vi "Event Handle Loop_Initialize.vi"(8 "error in (no error)":errorcluster, 11 "QMenu Class in":refnum<class "QMenu Class.lvclass">) -> (0 "error out":errorcluster, 3 "QMenu Class out":refnum<class "QMenu Class.lvclass">)   [LabVIEW 2020, in "QTab.lvlib" / "QMenu Class.lvclass"]
uses:
  QMenu Class.lvclass
  QMenu Class.lvclass/QMenu Class.ctl
  Read Left Button Image.vi
  Read Right Button Image.vi
  Read Close Button Image.vi
  Read Button Image.vi
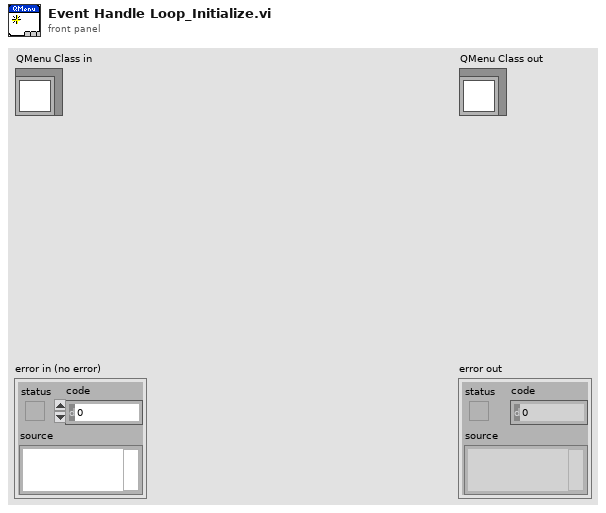
[diagram p1: front panel]
types:
  T1 = typedef "imagedata.ctl" = cluster{"image type":i32, "image depth":i32, "image":u8[], "mask":u8[], "colors":u32[], "Rectangle":cluster{"left":i16, "top":i16, "right":i16, "bottom":i16}}
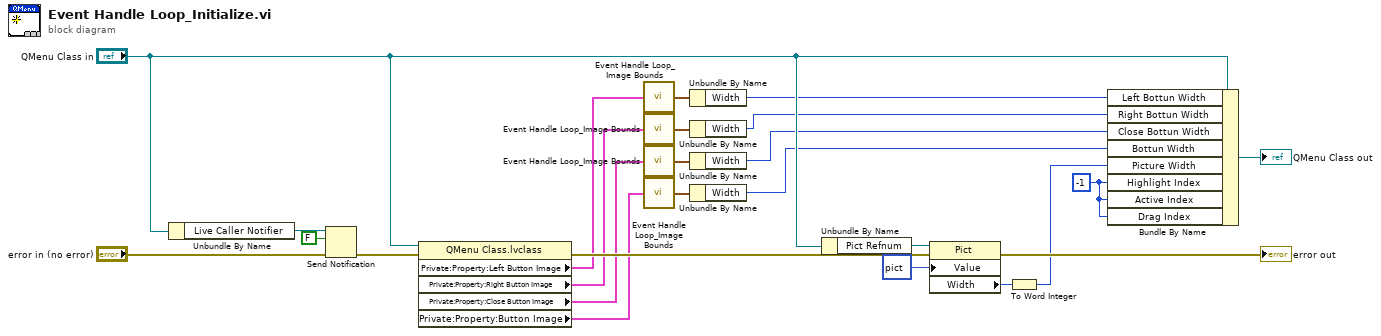
[diagram p0: block diagram]
diagram:
  w1 = -1 ("Buffer Data.Highlight Index")
  n1 = Unbundle By Name("QMenu Class in") -> ("Live Caller Notifier"=w24:refnum<notifier>)
  n2 = Send Notification(notification=FALSE ("element"), notifier=w24, error in (no error)="error in (no error)") -> (error out=w18:errorcluster)  [unwired: 1 out]
  n3 = property class="QMenu Class.lvclass"(reference="QMenu Class in", error in=w18) -> (error out=w16:errorcluster, "Private:Property:Left Button Image"=w14:T1, "Private:Property:Right Button Image"=w8:T1, "Private:Property:Close Button Image"=w7:T1, "Private:Property:Button Image"=w6:T1)  [unwired: 1 out]
  n4 = call "Event Handle Loop_Image Bounds.vi"("Image"=w14) -> ("Bounds"=w13:cluster{"Width":i16, "Height":i16})
  n5 = call "Event Handle Loop_Image Bounds.vi"("Image"=w8) -> ("Bounds"=w11:cluster{"Width":i16, "Height":i16})
  n6 = call "Event Handle Loop_Image Bounds.vi"("Image"=w7) -> ("Bounds"=w10:cluster{"Width":i16, "Height":i16})
  n7 = call "Event Handle Loop_Image Bounds.vi"("Image"=w6) -> ("Bounds"=w9:cluster{"Width":i16, "Height":i16})
  n8 = Unbundle By Name(w13) -> ("Width"=w12:i16)
  n9 = Unbundle By Name(w11) -> ("Width"=w5:i16)
  n10 = Unbundle By Name(w10) -> ("Width"=w4:i16)
  n11 = Unbundle By Name(w9) -> ("Width"=w3:i16)
  n12 = Unbundle By Name("QMenu Class in") -> ("Pict Refnum"=w22:refnum<vi>)
  n13 = property class="Pict"(reference=w22, error in=w16, "Value"=picture data[5B]) -> (error out=→"error out":errorcluster, "Width"=w20:u32)  [unwired: 1 out]
  n14 = To Word Integer(number=w20) -> (16bit integer=w2:i16)
  n15 = Bundle By Name(cluster="QMenu Class in", "Left Bottun Width"=w12, "Right Bottun Width"=w5, "Close Bottun Width"=w4, "Bottun Width"=w3, "Picture Width"=w2, "Highlight Index"=w1, "Active Index"=w1, "Drag Index"=w1) -> (→"QMenu Class out":refnum<class "QMenu Class.lvclass">)
